vi "backup_imp_test_v8.vi"() -> ()   [LabVIEW 2014]
uses:
  <vilib>/eio/EIOPropertyNode/EIOPropertyNode.xnode
  <vilib>/LabVIEW Targets/FPGA/cRIO/shared/nicrio_ModuleControls/nicrio_cRIO-9237_DataRatesRing.ctl
  <vilib>/LabVIEW Targets/FPGA/cRIO/shared/nicrio_ModuleControls/nicrio_cRIO-9237_ExcitationVoltageRing.ctl
  <vilib>/rvi/eio/common/nirviEmuTemplatePropertyGet_errors.vi
  <vilib>/rvi/eio/common/nirviEmuTemplatePropertyGet_noerrors.vi
  <vilib>/rvi/eio/common/nirviEmuTemplatePropertySet_errors.vi
  <vilib>/rvi/eio/common/nirviEmuTemplatePropertySet_noerrors.vi
  <vilib>/eio/EIONode/EIONode.xnode
  <vilib>/rvi/eio/common/nirviEmuTemplateMethod_errors.vi
  <vilib>/rvi/Analysis/measure/butterworth/XNode/niFpgaButterworthFilter.xnode
  <vilib>/rvi/DataTransferAndStorage/Container/XNode/niFpgaContainer.xnode
  <vilib>/rvi/FXPMathLib/FxpMul/XNode/nifxpmath_Multiplier.xnode
  <vilib>/rvi/FXPMathLib/sim/FxpSim.dll
  <vilib>/rvi/FXPMathLib/FxpSinAndCos/XNode/nifxpmath_SinAndCos.xnode
  <vilib>/rvi/FXPMathLib/FxpSinAndCos/simVIs/DllFxpSinAndCosTemp_sub.vi
  <vilib>/rvi/FXPMathLib/FxpSinAndCos/subVIs/nifxpmath_SinAndCos_SimConfig.ctl
  <vilib>/rvi/FXPMathLib/FxpSub/XNode/nifxpmath_Sub.xnode
  <vilib>/rvi/FXPMathLib/FxpAdd/XNode/nifxpmath_Add.xnode
  <vilib>/rvi/interface/RandomDataEmulation/nirviRandomDataFpgaMultiElementTemplate.vi
panel:
  out "omega_y (rad/s)":fxp<+/-,36,13>
  out "Dy_d (mm/s)":fxp<+/-,36,13>
  in  "Vy. Est.":i16(ring) items=["T", "Mavg"]
  out "omega_y (Mavg)":fxp<+/-,36,13>
  out "Dy_d (Mavg)":fxp<+/-,36,13>
  in  "Dy_d_M_avg_Tc (uSec)":i32 caption="Dp_d_M_avg_Tc (uSec)"
  out "Dp_d (Mavg)":fxp<+/-,36,13>
  out "omega_p (Mavg)":fxp<+/-,36,13>
  in  "Dp_d_M_avg_Tc (uSec)":i32
  out "Dp_d (T)":fxp<+/-,36,13>
  out "omega_p (T)":fxp<+/-,36,13>
  in  "Vp. Est.":i16(ring) items=["T", "Mavg"]
  in  "Mag. factor":fxp<+/-,20,3>
  in  "Mag. encoder_p":bool
  in  "Belt_op":fxp<+/-,7,7>
  in  "Belt_mp":fxp<+/-,6,6>
  in  "Belt_oy":fxp<+/-,7,7>
  in  "Belt_my":fxp<+/-,6,6>
  out "Fp_dc":fxp<+/-,32,10>
  out "Fy_dc":fxp<+/-,32,10>
  in  "Zero_y":bool
  in  "Zero_p":bool
  in  "mt0_omega_p":u32
  in  "Encoder reset":bool
  out "fpt_d":fxp<+/-,36,18>
  out "Dp_error_dd":fxp<+/-,36,16>
  out "Dp_error_d":fxp<+/-,33,8>
  in  "Dp_dd coeff.":i32[](array[numeric])=[946630756, 63555534]
  out "Dp_dd":fxp<+/-,36,25>
  out "dFp_PID":fxp<+/-,36,18>
  in  "dFp_PID coeff.":i32[](array[numeric])=[946630756, 63555534]
  out "fpt_i":fxp<+/-,34,18>
  in  "Bv_p":fxp<+/-,22,8>
  in  "Kv_p":fxp<+/-,22,8>
  out "Dp_error":fxp<+/-,22,7>
  out "Dpr_sin":fxp<+/-,22,7>
  in  "Sin offset_p":fxp<+/-,22,7>
  in  "Sin magnitude_p":fxp<+/-,21,6>
  out "Dpr_sin_dd":fxp<+/-,35,20>
  out "Dpr_sin_d":fxp<+/-,33,15>
  out "Sin omega_p":fxp<+/-,34,9>
  in  "Sin wave freq._p (Hz)":fxp<+/-,32,6>
  in  "Dpr_step":fxp<+/-,22,7>
  out "Dpr_for":fxp<+/-,22,7>
  in  "Command_p":i16(ring) items=["Step", "Sine"]
  in  "Ki_p":fxp<+/-,36,9>
  out "Fp_PID":fxp<+/-,36,16>
  in  "fp_tolorance":fxp<+,22,6>
  out "fp_tilde":fxp<+/-,33,10>
  in  "Kd_p":fxp<+/-,36,9>
  in  "Kp_p":fxp<+/-,36,9>
  out "Fr_p":fxp<+/-,32,10>
  in  "S/F coeff_p":fxp<+/-,25,-10>
  in  "S/F coeff_y":fxp<+/-,25,-10>
  out "va_p":fxp<+/-,36,7>
  out "vb_p":fxp<+/-,37,8>
  out "vq_p_F":fxp<+/-,20,5> format="%.57g"
  out "vd_p_F":fxp<+/-,20,5>
  in  "dFp_add":bool
  in  "Stop motor_p":bool
  out "Force_p":fxp<+/-,32,10>
  in  "Strain selection_p":i16(ring) items=["Raw", "Avg.8", "Avg.8 w. filter"]
  out "Strain_p (Avg8 w. f)":fxp<+/-,36,8>
  in  "Strain_p Avg.8 coeff.":i32[](array[numeric])=[946630756, 63555534]
  out "Strain_p (Avg8)":fxp<+/-,36,4>
  out "Raw Strain_p":fxp<+/-,36,4>
  out "Mod6/AI3":fxp<+/-,36,4>
  in  "Strain gage reset_p":bool
  out "Dp_d (mm/s)":fxp<+/-,36,13>
  out "omega_p (rad/s)":fxp<+/-,36,13>
  out "mt_omega_p":u32
  out "rad_p(NrTheta)":fxp<+/-,33,20>
  out "D_p(mm)":fxp<+/-,32,7>
  out "Encoder Position_p":i32
  in  "Encoder reset_p":bool
  out "Strain_y (Avg8 w. f)":fxp<+/-,36,8>
  in  "Strain_y Avg8 coeff.":i32[](array[numeric])=[-898916953, 1957103773, 3888751]
  out "Dyr_for":fxp<+/-,22,7>
  in  "Command_y":i16(ring) items=["Step", "Sine"]
  out "Strain_y (Avg8)":fxp<+/-,36,4>
  in  "Strain selection_y":i16(ring) items=["Raw", "Avg.8", "Avg.8 w. filter"]
  out "vb_y":fxp<+/-,38,8>
  out "va_y":fxp<+/-,38,8>
  out "fyt_d":fxp<+/-,36,18>
  out "Fr_y":fxp<+/-,32,10>
  in  "Bv_y":fxp<+/-,22,8>
  out "Dy_error_dd":fxp<+/-,36,16>
  out "Dy_error_d":fxp<+/-,33,8>
  in  "Kv_y":fxp<+/-,22,8>
  out "Dy_error":fxp<+/-,22,7>
  out "Dyr_sin_dd":fxp<+/-,35,20>
  out "Dyr_sin_d":fxp<+/-,33,15>
  out "Sin omega_y":fxp<+/-,34,9>
  out "Dyr_sin":fxp<+/-,22,7>
  in  "Sin offset_y":fxp<+/-,22,7>
  in  "Sin magnitude_y":fxp<+/-,21,6>
  out "Time now(s)":fxp<+,52,14>
  in  "Sin wave freq._y (Hz)":fxp<+/-,32,6>
  in  "Dyr_step":fxp<+/-,22,7>
  in  "Drive mode":i16(ring) items=["Backward", "Forward"]
  out "Dy_dd":fxp<+/-,36,25>
  in  "Dy_dd coeff.":i32[](array[numeric])=[946630756, 63555534]
  out "dFy_PID":fxp<+/-,36,18>
  in  "dFy_PID coeff.":i32[](array[numeric])=[946630756, 63555534]
  out "fyt_i":fxp<+/-,36,16>
  out "Fy_PID":fxp<+/-,36,16>
  in  "fy_tolorance":fxp<+,22,6>
  in  "Ki_y":fxp<+/-,36,9>
  in  "Kd_y":fxp<+/-,36,9>
  out "fy_tilde":fxp<+/-,32,10>
  in  "Kp_y":fxp<+/-,36,9>
  out "vq_y_F":fxp<+/-,20,5> format="%.57g"
  out "vd_y_F":fxp<+/-,20,5>
  in  "dFy_add":bool
  in  "Stop motor_y":bool
  out "Dy_d (T)":fxp<+/-,36,13>
  out "omega_y (T)":fxp<+/-,36,13>
  in  "mt0_omega_y":u32
  out "mt_omega_y":u32
  out "rad_y(NrTheta)":fxp<+/-,33,20>
  out "D_y(mm)":fxp<+/-,32,7>
  out "Encoder Position_y":i32
  in  "Encoder reset_y":bool
  in  "Ini coe.":bool
  out "Loop rate (kHz)":fxp<+/-,36,7>
  out "Force_y":fxp<+/-,32,10>
  out "Raw Strain_y":fxp<+/-,36,4>
  in  "Strain gage reset_y":bool
  in  "Stop (Strain)":bool
  out "Mod6/AI2":fxp<+/-,36,4>
  in  "Excitation Voltage":T1 items=["2.5 Volts", "3.3 Volts", "5.0 Volts", "10.0 Volts", "External Excitation"]
  in  "Data Rate":T2=1 items=["50.000 kS/s (NI 9237)"=1, "25.000 kS/s (NI 9237)"=2, "16.667 kS/s (NI 9237)"=3, "12.500 kS/s (NI 9237)"=4, "10.000 kS/s (NI 9237)"=5, "8.333 kS/s (NI 9237)"=6, "7.143 kS/s (NI 9237)"=7, "6.250 kS/s (NI 9237)"=8, "5.556 kS/s (NI 9237)"=9, "5.000 kS/s (NI 9237)"=10, "4.545 kS/s (NI 9237)"=11, "4.167 kS/s (NI 9237)"=12, "3.846 kS/s (NI 9237)"=13, "3.571 kS/s (NI 9237)"=14, "3.333 kS/s (NI 9237)"=15, "3.125 kS/s (NI 9237)"=16, "2.941 kS/s (NI 9237)"=17, "2.778 kS/s (NI 9237)"=18, "2.632 kS/s (NI 9237)"=19, "2.500 kS/s (NI 9237)"=20, "2.381 kS/s (NI 9237)"=21, "2.273 kS/s (NI 9237)"=22, "2.174 kS/s (NI 9237)"=23, "2.083 kS/s (NI 9237)"=24, "2.000 kS/s (NI 9237)"=25, "1.923 kS/s (NI 9237)"=26, "1.852 kS/s (NI 9237)"=27, "1.786 kS/s (NI 9237)"=28, "1.724 kS/s (NI 9237)"=29, "1.667 kS/s (NI 9237)"=30, "1.613 kS/s (NI 9237)"=31]
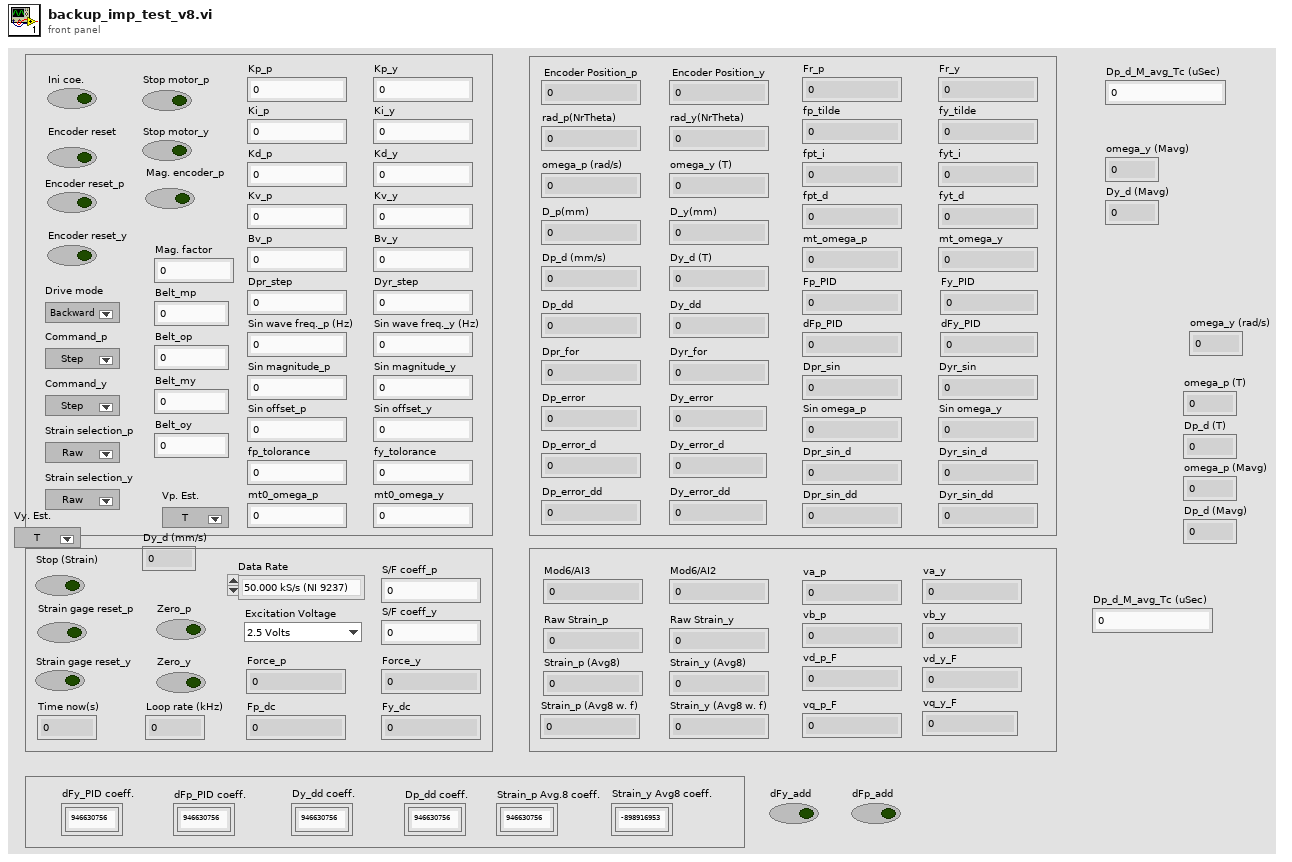
[diagram p1: front panel]
types:
  T1 = typedef "nicrio_cRIO-9237_ExcitationVoltageRing.ctl" = u8
  T2 = typedef "nicrio_cRIO-9237_DataRatesRing.ctl" = u8
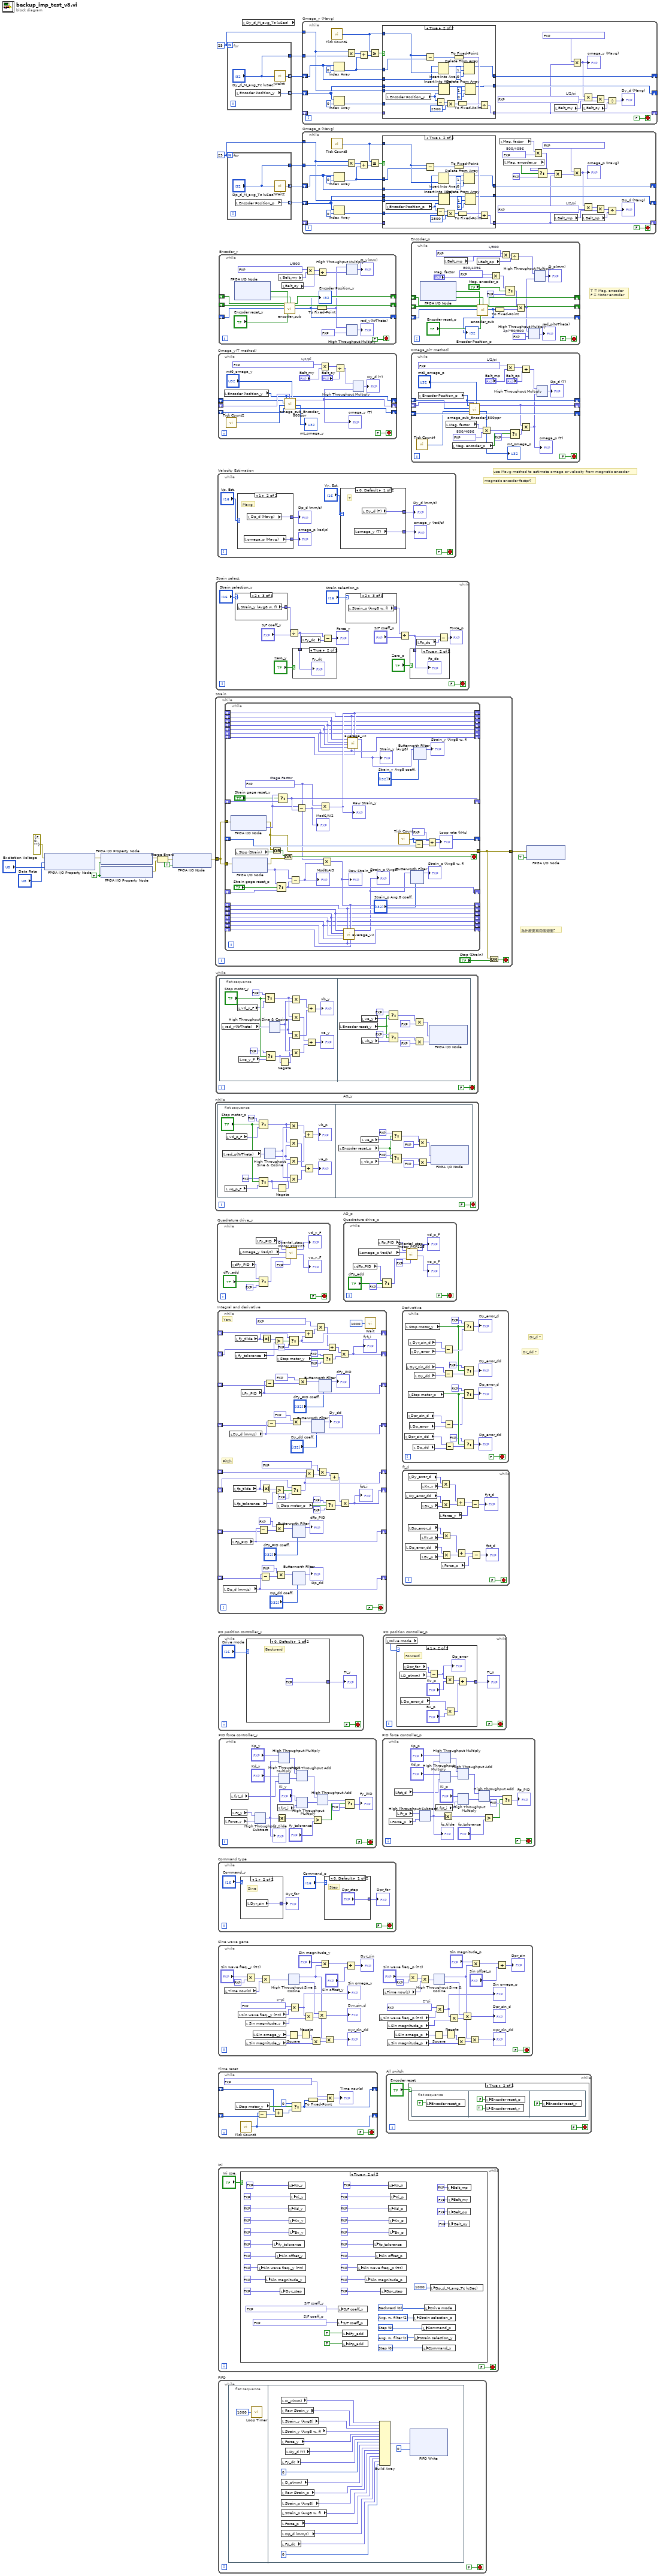
[diagram p0: block diagram]
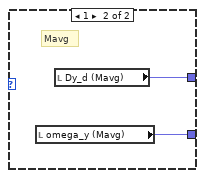
[diagram p4: hidden frame]
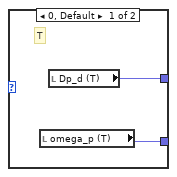
[diagram p5: hidden frame]
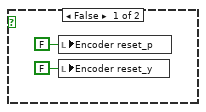
[diagram p6: hidden frame]
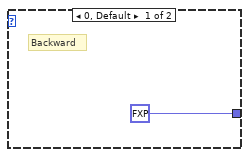
[diagram p7: hidden frame]
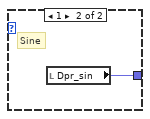
[diagram p8: hidden frame]
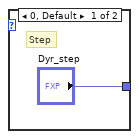
[diagram p9: hidden frame]
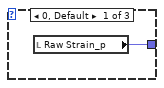
[diagram p12: hidden frame]
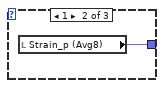
[diagram p13: hidden frame]
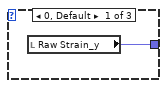
[diagram p14: hidden frame]
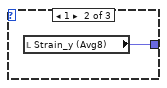
[diagram p15: hidden frame]
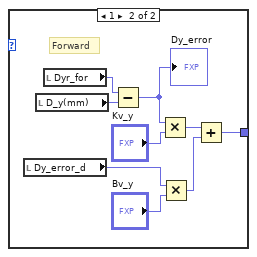
[diagram p16: hidden frame]
diagram:
  w5 = 25
  w8 = 25
  w13 = TRUE ("Half-Bridge Enable")
  # "use Mavg method to estimate omega or velocity from magnetic encoder"
  # "T = Mag. encoder\nF = Motor encoder"
  # "magnetic encoder factpr?"
  # "為什麼要寫兩個迴圈?"
  # "Dr_dd ?"
  # "Dr_d ?"
  n1 = xnode "FPGA I/O Property Node"("error in"=errorcluster {"status"=FALSE, "code"=0, "source"=""}, "Data Rate"="Data Rate", "Excitation Voltage"="Excitation Voltage") -> ("error out"=w18:errorcluster)  [unwired: 1 in, 1 out]
  n2 = xnode "FPGA I/O Property Node"("error in"=w18, "Half-Bridge Enable"=w13) -> ("error out"=w11:errorcluster)  [unwired: 1 in, 1 out]
  n3 = xnode "FPGA I/O Property Node"("Half-Bridge Enable"=w13) -> ("error out"=w10:errorcluster)  [unwired: 2 in, 1 out]
  n4 = Merge Errors(w11, w10) -> (w12:errorcluster)
  n5 = xnode "FPGA I/O Node"("error in"=w12, "Mod6/Start"=TRUE) -> ("error out"=w16:errorcluster)  [unwired: 1 in, 1 out]
  n6 = while "Strain" {
    tunnel: w16 -> [w23]
    tunnel: [w21] -> w9
    stop <- w22 stop-if-true
    n7 = while {
      tunnel: w23 -> [w69]
      tunnel: [w42] -> w21
      shift-right: [w66] -> _
      shift-left: _ -> [w67]
      shift-right: [w62] -> _
      shift-left: _ -> [w63]
      shift-right: [w57] -> _
      shift-left: _ -> [w56]
      shift-right: [w56] -> _
      shift-left: _ -> [w55]
      shift-right: [w55] -> _
      shift-left: _ -> [w54]
      shift-right: [w54] -> _
      shift-left: _ -> [w53]
      shift-right: [w53] -> _
      shift-left: _ -> [w52]
      shift-right: [w52] -> _
      shift-left: _ -> [w51]
      shift-right: [w51] -> _
      shift-left: _ -> [w50]
      tunnel: w23 -> [w46]
      shift-right: [w39] -> _
      shift-left: _ -> [w40]
      shift-right: [w35] -> _
      shift-left: _ -> [w34]
      shift-right: [w34] -> _
      shift-left: _ -> [w33]
      shift-right: [w33] -> _
      shift-left: _ -> [w32]
      shift-right: [w32] -> _
      shift-left: _ -> [w31]
      shift-right: [w31] -> _
      shift-left: _ -> [w30]
      shift-right: [w30] -> _
      shift-left: _ -> [w29]
      shift-right: [w29] -> _
      shift-left: _ -> [w28]
      stop <- w43 stop-if-true
      w37 = fxp<+,20,2> 2.115001678466797  # Gage Factor
      n8 = xnode "FPGA I/O Node"("error in"=w69) -> ("error out"=w42:errorcluster, "Mod6/AI2"=w64:fxp<+/-,24,-4>)  [unwired: 1 in, 1 out]
      n9 = xnode "FPGA I/O Node"("error in"=w46) -> ("error out"=w44:errorcluster, "Mod6/AI3"=w38:fxp<+/-,24,-4>)  [unwired: 1 in, 1 out]
      n10 = local read "Stop (Strain)"() -> (w68:bool)
      n11 = Or(x=w42, y=w68) -> (x .or. y?=w45:bool)
      n12 = Select(t=w38, s="Strain gage reset_p", f=w40) -> (s? t:f=w39:fxp<+/-,24,-4>)
      n13 = Select(t=w64, s="Strain gage reset_y", f=w67) -> (s? t:f=w66:fxp<+/-,24,-4>)
      n14 = Or(x=w45, y=w44) -> (x .or. y?=w43:bool)
      n15 = Subtract(x=w38, y=w39) -> (x-y=w36:fxp<+/-,30,-3>)
      "Mod6/AI3" <- w36
      n16 = Subtract(x=w64, y=w66) -> (x-y=w65:fxp<+/-,30,-3>)
      "Mod6/AI2" <- w65
      n17 = Multiply(x=w37, y=w65) -> (x*y=w57:fxp<+/-,41,6>)
      "Raw Strain_y" <- w57
      n18 = Multiply(x=w37, y=w36) -> (x*y=w35:fxp<+/-,50,-1>)
      "Raw Strain_p" <- w35
      n19 = call "average_v2.vi"("Numeric 8"=w28, "Numeric"=w35, "Numeric 7"=w29, "Numeric 2"=w34, "Numeric 6"=w30, "Numeric 5"=w31, "Numeric 4"=w32, "Numeric 3"=w33) -> ("Mean (8pt)"=w27:fxp<+/-,32,4>)  [unwired: 1 in, 2 out]
      "Strain_p (Avg8)" <- w27
      n20 = call "average_v2.vi"("Numeric 8"=w50, "Numeric"=w57, "Numeric 7"=w51, "Numeric 2"=w56, "Numeric 6"=w52, "Numeric 5"=w53, "Numeric 4"=w54, "Numeric 3"=w55) -> ("Mean (8pt)"=w49:fxp<+/-,32,4>)  [unwired: 1 in, 2 out]
      "Strain_y (Avg8)" <- w49
      n21 = call "Tick Count"() -> ("Tick Count(uSec)"=w62:u32)
      n22 = xnode "Butterworth Filter"("input data"=w27, "scaled coefficients"="Strain_p Avg.8 coeff.") -> ("output data"=→"Strain_p (Avg8 w. f)":fxp<+/-,36,8>)  [unwired: 1 in]
      n23 = xnode "Butterworth Filter"("input data"=w49, "scaled coefficients"="Strain_y Avg8 coeff.") -> ("output data"=→"Strain_y (Avg8 w. f)":fxp<+/-,32,4>)  [unwired: 1 in]
      n24 = Subtract(x=w62, y=w63) -> (x-y=w60:fxp<+/-,32,16>)
      n25 = Divide(x=fxp<+,7,10> 1000.0, y=w60) -> (x/y=→"Loop rate (kHz)":fxp<+/-,40,27>)
    }
    n26 = Or(x=w21, y="Stop (Strain)") -> (x .or. y?=w22:bool)
  }
  n27 = while "AO_p" {
    stop <- FALSE stop-if-true
    n28 = flat-sequence {
      frame #0 {
        n29 = local read "rad_p(NrTheta)"() -> (w98:fxp<+/-,33,20>)
        n30 = local read "vq_p_F"() -> (w99:fxp<+/-,20,5>)
        n31 = local read "vd_p_F"() -> (w101:fxp<+/-,20,5>)
        n32 = Select(t=fxp<+/-,20,5> 0.0, s="Stop motor_p", f=w101) -> (s? t:f=w90:fxp<+/-,20,5>)
        n33 = Select(t=fxp<+,1,1> 0.0, s="Stop motor_p", f=w99) -> (s? t:f=w89:fxp<+/-,20,5>)
        n34 = xnode "High Throughput Sine & Cosine"("x (pi)"=w98) -> ("sin(x)"=w92:fxp<+/-,16,2>, "cos(x)"=w91:fxp<+/-,16,2>)
        n35 = Negate(x=w89) -> (-x=w97:fxp<+/-,21,6>)
        n36 = Multiply(x=w90, y=w92) -> (x*y=w96:fxp<+/-,36,7>)
        n37 = Multiply(x=w90, y=w91) -> (x*y=w94:fxp<+/-,36,7>)
        n38 = Multiply(x=w91, y=w89) -> (x*y=w95:fxp<+/-,36,7>)
        n39 = Multiply(x=w92, y=w97) -> (x*y=w93:fxp<+/-,35,6>)
        n40 = Add(x=w96, y=w95) -> (x+y=→"vb_p":fxp<+/-,37,8>)
        n41 = Add(x=w94, y=w93) -> (x+y=→"va_p":fxp<+/-,36,7>)
      }
      frame #1 {
        n42 = local read "Encoder reset_p"() -> (w134:bool)
        n43 = local read "vb_p"() -> (w135:fxp<+/-,37,8>)
        n44 = local read "va_p"() -> (w136:fxp<+/-,36,7>)
        n45 = Select(t=fxp<+,2,2> 3.0, s=w134, f=w136) -> (s? t:f=w142:fxp<+/-,36,7>)
        n46 = Select(t=fxp<+,1,1> 0.0, s=w134, f=w135) -> (s? t:f=w141:fxp<+/-,37,8>)
        n47 = Multiply(x=w142, y=fxp<+/-,1,0> -0.5) -> (x*y=w137:fxp<+/-,36,6>)
        n48 = Multiply(x=w141, y=fxp<+/-,1,0> -0.5) -> (x*y=w138:fxp<+/-,36,6>)
        n49 = xnode "FPGA I/O Node"("Mod8/AO0"=w137, "Mod8/AO1"=w138) -> ()  [unwired: 2 in, 2 out]
      }
    }
  }
  n50 = while "AO_y" {
    stop <- FALSE stop-if-true
    n51 = flat-sequence {
      frame #0 {
        n52 = local read "rad_y(NrTheta)"() -> (w162:fxp<+/-,33,20>)
        n53 = local read "vd_y_F"() -> (w160:fxp<+/-,20,5>)
        n54 = local read "vq_y_F"() -> (w159:fxp<+/-,20,5>)
        n55 = Select(t=fxp<+/-,20,5> 0.0, s="Stop motor_y", f=w160) -> (s? t:f=w154:fxp<+/-,20,5>)
        n56 = Select(t=fxp<+/-,20,5> 0.0, s="Stop motor_y", f=w159) -> (s? t:f=w153:fxp<+/-,20,5>)
        n57 = xnode "High Throughput Sine & Cosine"("x (pi)"=w162) -> ("sin(x)"=w156:fxp<+/-,17,2>, "cos(x)"=w155:fxp<+/-,17,2>)
        n58 = Negate(x=w153) -> (-x=w152:fxp<+/-,21,6>)
        n59 = Multiply(x=w154, y=w156) -> (x*y=w151:fxp<+/-,37,7>)
        n60 = Multiply(x=w154, y=w155) -> (x*y=w149:fxp<+/-,37,7>)
        n61 = Multiply(x=w155, y=w153) -> (x*y=w150:fxp<+/-,37,7>)
        n62 = Multiply(x=w156, y=w152) -> (x*y=w148:fxp<+/-,36,6>)
        n63 = Add(x=w151, y=w150) -> (x+y=→"vb_y":fxp<+/-,38,8>)
        n64 = Add(x=w149, y=w148) -> (x+y=→"va_y":fxp<+/-,37,7>)
      }
      frame #1 {
        n65 = local read "Encoder reset_y"() -> (w195:bool)
        n66 = local read "va_y"() -> (w194:fxp<+/-,38,8>)
        n67 = local read "vb_y"() -> (w193:fxp<+/-,38,8>)
        n68 = Select(t=fxp<+,2,2> 3.0, s=w195, f=w194) -> (s? t:f=w199:fxp<+/-,38,8>)
        n69 = Select(t=fxp<+,1,1> 0.0, s=w195, f=w193) -> (s? t:f=w198:fxp<+/-,38,8>)
        n70 = Multiply(x=w199, y=fxp<+/-,1,0> -0.5) -> (x*y=w202:fxp<+/-,39,8>)
        n71 = Multiply(x=w198, y=fxp<+/-,1,0> -0.5) -> (x*y=w203:fxp<+/-,37,6>)
        n72 = xnode "FPGA I/O Node"("Mod8/AO2"=w202, "Mod8/AO3"=w203) -> ()  [unwired: 2 in, 2 out]
      }
    }
  }
  n73 = while "Strain select." {
    stop <- FALSE stop-if-true
    n74 = case shown="2" "Strain selection_y" {
      tunnel: [w224 w225 w226] -> w217
      frame 0, Default {
        n75 = local read "Raw Strain_y"() -> (w224:fxp<+/-,36,4>)
      }
      frame 1 {
        n76 = local read "Strain_y (Avg8)"() -> (w225:fxp<+/-,36,4>)
      }
      frame 2 {
        n77 = local read "Strain_y (Avg8 w. f)"() -> (w226:fxp<+/-,36,8>)
      }
    }
    n78 = Divide(x=w217, y="S/F coeff_y") -> (x/y=w210:fxp<+/-,32,10>)
    n79 = case shown="True" "Zero_y" {
      tunnel: w210 -> [_ w220]
      frame False {
      }
      frame True {
        "Fy_dc" <- w220
      }
    }
    n80 = local read "Fy_dc"() -> (w211:fxp<+/-,32,10>)
    n81 = Subtract(x=w210, y=w211) -> (x-y=→"Force_y":fxp<+/-,33,11>)
    n82 = case shown="2" "Strain selection_p" {
      tunnel: [w221 w222 w223] -> w215
      frame 0, Default {
        n83 = local read "Raw Strain_p"() -> (w221:fxp<+/-,36,4>)
      }
      frame 1 {
        n84 = local read "Strain_p (Avg8)"() -> (w222:fxp<+/-,36,4>)
      }
      frame 2 {
        n85 = local read "Strain_p (Avg8 w. f)"() -> (w223:fxp<+/-,36,8>)
      }
    }
    n86 = Divide(x=w215, y="S/F coeff_p") -> (x/y=w207:fxp<+/-,32,10>)
    n87 = case shown="True" "Zero_p" {
      tunnel: w207 -> [_ w219]
      frame False {
      }
      frame True {
        "Fp_dc" <- w219
      }
    }
    n88 = local read "Fp_dc"() -> (w205:fxp<+/-,32,10>)
    n89 = Subtract(x=w207, y=w205) -> (x-y=→"Force_p":fxp<+/-,33,11>)
  }
  n90 = while "Quadrature drive_y" {
    stop <- FALSE stop-if-true
    n91 = local read "dFy_PID"() -> (w228:fxp<+/-,36,18>)
    n92 = local read "omega_y (rad/s)"() -> (w236:fxp<+/-,36,13>)
    n93 = local read "Fy_PID"() -> (w229:fxp<+/-,36,16>)
    n94 = Select(t=w228, s="dFy_add", f=fxp<+,1,1> 0.0) -> (s? t:f=w232:fxp<+/-,36,18>)
    n95 = call "Oriental_step_motor_PKP225.vi"("F_Threshold"=fxp<+,12,12> 10.0, "dFmr"=w232, "omega"=w236, "Fmr"=w229) -> ("vq_F"=→"vq_y_F":fxp<+/-,20,5>, "vd_F"=→"vd_y_F":fxp<+/-,20,5>)  [unwired: 6 in]
  }
  n96 = while "Integral and derivative" {
    shift-right: [w292] -> _
    shift-left: _ -> [w291]
    shift-right: [w284] -> _
    shift-left: _ -> [w283]
    shift-right: [w294] -> _
    shift-left: _ -> [w295]
    shift-right: [w274] -> _
    shift-left: _ -> [w273]
    shift-right: [w260] -> _
    shift-left: _ -> [w263]
    shift-right: [w253] -> _
    shift-left: _ -> [w252]
    shift-right: [w247] -> _
    shift-left: _ -> [w246]
    shift-right: [w242] -> _
    shift-left: _ -> [w243]
    stop <- FALSE stop-if-true
    # "Pitch"
    # "Yaw"
    n97 = local read "Dp_d (mm/s)"() -> (w242:fxp<+/-,36,13>)
    n98 = local read "Dy_d (mm/s)"() -> (w274:fxp<+/-,36,13>)
    n99 = local read "Fp_PID"() -> (w247:fxp<+/-,36,16>)
    n100 = local read "fp_tilde"() -> (w264:fxp<+/-,33,10>)
    n101 = local read "fp_tolorance"() -> (w267:fxp<+,22,6>)
    n102 = local read "fy_tolorance"() -> (w270:fxp<+,22,6>)
    n103 = local read "fy_tilde"() -> (w296:fxp<+/-,32,10>)
    n104 = local read "Fy_PID"() -> (w294:fxp<+/-,36,16>)
    n105 = Subtract(x=w247, y=w246) -> (x-y=w251:fxp<+/-,37,17>)
    n106 = Subtract(x=w242, y=w243) -> (x-y=w244:fxp<+/-,37,14>)
    n107 = Absolute Value(x=w264) -> (abs(x)=w268:fxp<+,33,10>)
    n108 = Absolute Value(x=w296) -> (abs(x)=w298:fxp<+,32,10>)
    n109 = Subtract(x=w294, y=w295) -> (x-y=w282:fxp<+/-,37,17>)
    n110 = Subtract(x=w274, y=w273) -> (x-y=w276:fxp<+/-,36,11>)
    n111 = Greater?(x=w298, y=w270) -> (0:w299:bool)
    n112 = Greater?(x=w268, y=w267) -> (0:w266:bool)
    n113 = Multiply(x=fxp<+,7,10> 1000.0, y=w251) -> (x*y=w249:fxp<+/-,32,18>)
    n114 = Multiply(x=fxp<+,7,10> 1000.0, y=w244) -> (x*y=w240:fxp<+/-,36,21>)
    n115 = local read "Stop motor_y"() -> (w285:bool)
    n116 = local read "Stop motor_p"() -> (w255:bool)
    n117 = Select(t=w296, s=w299, f=fxp<+/-,33,11> 0.0) -> (s? t:f=w292:fxp<+/-,33,11>)
    n118 = Select(t=w264, s=w266, f=fxp<+,1,1> 0.0) -> (s? t:f=w260:fxp<+/-,33,10>)
    n119 = Multiply(x=fxp<+,7,10> 1000.0, y=w276) -> (x*y=w275:fxp<+/-,36,21>)
    n120 = xnode "Butterworth Filter"("input data"=w249, "scaled coefficients"="dFp_PID coeff.") -> ("output data"=→"dFp_PID":fxp<+/-,36,22>)  [unwired: 1 in]
    n121 = xnode "Butterworth Filter"("input data"=w240, "scaled coefficients"="Dp_dd coeff.") -> ("output data"=→"Dp_dd":fxp<+/-,36,25>)  [unwired: 1 in]
    n122 = Multiply(x=fxp<+,7,10> 1000.0, y=w282) -> (x*y=w279:fxp<+/-,32,18>)
    n123 = Add(x=w291, y=w292) -> (x+y=w297:fxp<+/-,34,12>)
    n124 = Multiply(x=w263, y=w260) -> (x*y=w262:fxp<+/-,34,12>)
    n125 = xnode "Butterworth Filter"("input data"=w275, "scaled coefficients"="Dy_dd coeff.") -> ("output data"=→"Dy_dd":fxp<+/-,36,25>)  [unwired: 1 in]
    n126 = Multiply(x=fxp<+/-,30,12> 0.000499725341796875, y=w297) -> (x*y=w290:fxp<+/-,34,10>)
    n127 = Multiply(x=fxp<+/-,30,12> 0.000499725341796875, y=w262) -> (x*y=w259:fxp<+/-,34,10>)
    n128 = xnode "Butterworth Filter"("input data"=w279, "scaled coefficients"="dFy_PID coeff.") -> ("output data"=→"dFy_PID":fxp<+/-,36,22>)  [unwired: 1 in]
    n129 = Select(t=fxp<+,1,1> 0.0, s=w285, f=fxp<+,1,1> 1.0) -> (s? t:f=w288:fxp<+,1,1>)
    n130 = Select(t=fxp<+,1,1> 0.0, s=w255, f=fxp<+,1,1> 1.0) -> (s? t:f=w257:fxp<+,1,1>)
    n131 = Add(x=w290, y=w283) -> (x+y=w289:fxp<+/-,36,16>)
    n132 = Add(x=w259, y=w252) -> (x+y=w258:fxp<+/-,36,16>)
    n133 = Multiply(x=w289, y=w288) -> (x*y=w284:fxp<+/-,34,18>)
    "fyt_i" <- w284
    n134 = Multiply(x=w258, y=w257) -> (x*y=w253:fxp<+/-,34,18>)
    "fpt_i" <- w253
    n135 = call "Wait"("Count(uSec)"=u32 1000) -> ()  [unwired: 1 out]
  }
  n136 = while "Velocity Estimation" {
    stop <- FALSE stop-if-true
    n137 = case shown="1" "Vp. Est." {
      tunnel: [w345 w346] -> w338
      tunnel: [w344 w347] -> w337
      frame 0, Default {
        # "T"
        n138 = local read "omega_p (T)"() -> (w345:fxp<+/-,36,13>)
        n139 = local read "Dp_d (T)"() -> (w344:fxp<+/-,36,13>)
      }
      frame 1 {
        # "Mavg"
        n140 = local read "omega_p (Mavg)"() -> (w346:fxp<+/-,36,13>)
        n141 = local read "Dp_d (Mavg)"() -> (w347:fxp<+/-,36,13>)
      }
    }
    "Dp_d (mm/s)" <- w337
    "omega_p (rad/s)" <- w338
    n142 = case shown="0, Default" "Vy. Est." {
      tunnel: [w341 w343] -> w335
      tunnel: [w340 w342] -> w334
      frame 0, Default {
        # "T"
        n143 = local read "omega_y (T)"() -> (w340:fxp<+/-,36,13>)
        n144 = local read "Dy_d (T)"() -> (w341:fxp<+/-,36,13>)
      }
      frame 1 {
        # "Mavg"
        n145 = local read "omega_y (Mavg)"() -> (w342:fxp<+/-,36,13>)
        n146 = local read "Dy_d (Mavg)"() -> (w343:fxp<+/-,36,13>)
      }
    }
    "Dy_d (mm/s)" <- w335
    "omega_y (rad/s)" <- w334
  }
  n147 = while "Omega_y(T method)" {
    shift-right: [w355] -> _
    shift-left: _ -> [w356]
    shift-right: [w349] -> _
    shift-left: _ -> [w359]
    shift-right: [w361] -> _
    shift-left: _ -> [w362]
    stop <- FALSE stop-if-true
    w354 = fxp<+/-,32,0> 0.3183098859153688  # L/2/pi
    n148 = local read "Encoder Position_y"() -> (w355:i32)
    n149 = call "Tick Count2"() -> ("Tick Count(Ticks)"=w363:u32)
    n150 = call "omega_sub_Encoder_800ppr.vi"("mt0"="mt0_omega_y", "omega_pre"=w359, "ticks_m_pre"=w362, "ticks"=w363, "count_pre"=w356, "count"=w355) -> ("ticks_m"=w361:u32, "mt"=→"mt_omega_y":u32, "omega"=w349:fxp<+/-,36,13>)  [unwired: 3 in]
    "omega_y (T)" <- w349
    n151 = Multiply(x=w354, y="Belt_my") -> (x*y=w352:fxp<+/-,38,6>)
    n152 = Divide(x=w352, y="Belt_oy") -> (x/y=w350:fxp<+/-,20,1>)
    n153 = xnode ("High Throughput Multiply")("x"=w350, "y"=w349) -> ("x*y"=→"Dy_d (T)":fxp<+/-,56,14>)
  }
  n154 = while "PD position controller_y" {
    stop <- FALSE stop-if-true
    n155 = case shown="0, Default" "Drive mode" {
      tunnel: [fxp<+/-,62,19> 0.0 w369] -> w365
      frame 0, Default {
        # "Backward"
      }
      frame 1 {
        # "Forward"
        n156 = local read "Dy_error_d"() -> (w371:fxp<+/-,33,8>)
        n157 = local read "D_y(mm)"() -> (w376:fxp<+/-,32,7>)
        n158 = local read "Dyr_for"() -> (w368:fxp<+/-,22,7>)
        n159 = Subtract(x=w368, y=w376) -> (x-y=w375:fxp<+/-,33,8>)
        "Dy_error" <- w375
        n160 = Multiply(x=w375, y="Kv_y") -> (x*y=w373:fxp<+/-,54,15>)
        n161 = Multiply(x=w371, y="Bv_y") -> (x*y=w370:fxp<+/-,55,16>)
        n162 = Add(x=w373, y=w370) -> (x+y=w369:fxp<+/-,55,16>)
      }
    }
    "Fr_y" <- w365
  }
  n163 = while "Command type" {
    stop <- FALSE stop-if-true
    n164 = case shown="1" "Command_y" {
      tunnel: ["Dyr_step" w385] -> w380
      frame 0, Default {
        # "Step"
      }
      frame 1 {
        # "Sine"
        n165 = local read "Dyr_sin"() -> (w385:fxp<+/-,22,7>)
      }
    }
    "Dyr_for" <- w380
    n166 = case shown="0, Default" "Command_p" {
      tunnel: ["Dpr_step" w383] -> w378
      frame 0, Default {
        # "Step"
      }
      frame 1 {
        # "Sine"
        n167 = local read "Dpr_sin"() -> (w383:fxp<+/-,22,7>)
      }
    }
    "Dpr_for" <- w378
  }
  n168 = while "Sine wave gene" {
    stop <- FALSE stop-if-true
    w391 = fxp<+,20,3> 6.2831878662109375  # 2*pi
    w423 = fxp<+,20,3> 6.2831878662109375  # 2*pi
    n169 = local read "Time now(s)"() -> (w429:fxp<+,52,14>)
    n170 = local read "Sin wave freq._y (Hz)"() -> (w422:fxp<+/-,32,6>)
    n171 = Multiply(x="Sin wave freq._y (Hz)", y=fxp<+/-,10,3> 2.0) -> (x*y=w430:fxp<+/-,41,9>)
    n172 = local read "Sin magnitude_y"() -> (w420:fxp<+/-,21,6>)
    n173 = local read "Sin magnitude_y"() -> (w413:fxp<+/-,21,6>)
    n174 = local read "Sin omega_y"() -> (w416:fxp<+/-,34,9>)
    n175 = Multiply(x=w430, y=w429) -> (x*y=w428:fxp<+/-,41,19>)
    n176 = Square(x=w416) -> (x^2=w415:fxp<+,34,18>)
    n177 = xnode "High Throughput Sine & Cosine"("x (pi)"=w428) -> ("sin(x)"=w410:fxp<+/-,16,2>, "cos(x)"=w418:fxp<+/-,16,2>)
    n178 = Multiply(x=w423, y=w422) -> (x*y=w421:fxp<+/-,34,9>)
    "Sin omega_y" <- w421
    n179 = Negate(x=w415) -> (-x=w414:fxp<+/-,35,19>)
    n180 = Multiply(x=w421, y=w420) -> (x*y=w419:fxp<+/-,33,15>)
    n181 = Multiply(x=w414, y=w413) -> (x*y=w412:fxp<+/-,34,20>)
    n182 = Multiply(x=w418, y=w419) -> (x*y=→"Dyr_sin_d":fxp<+/-,33,15>)
    n183 = Multiply(x="Sin magnitude_y", y=w410) -> (x*y=w426:fxp<+/-,37,8>)
    n184 = Multiply(x=w410, y=w412) -> (x*y=→"Dyr_sin_dd":fxp<+/-,35,20>)
    n185 = Add(x=w426, y="Sin offset_y") -> (x+y=→"Dyr_sin":fxp<+/-,37,8>)
    n186 = local read "Sin wave freq._p (Hz)"() -> (w387:fxp<+/-,32,6>)
    n187 = local read "Time now(s)"() -> (w405:fxp<+,52,14>)
    n188 = local read "Sin magnitude_p"() -> (w388:fxp<+/-,21,6>)
    n189 = local read "Sin magnitude_p"() -> (w390:fxp<+/-,21,6>)
    n190 = local read "Sin omega_p"() -> (w389:fxp<+/-,34,9>)
    n191 = Multiply(x="Sin wave freq._p (Hz)", y=fxp<+/-,10,3> 2.0) -> (x*y=w409:fxp<+/-,42,9>)
    n192 = Multiply(x=w409, y=w405) -> (x*y=w406:fxp<+/-,41,19>)
    n193 = Square(x=w389) -> (x^2=w401:fxp<+,34,18>)
    n194 = xnode "High Throughput Sine & Cosine"("x (pi)"=w406) -> ("sin(x)"=w392:fxp<+/-,16,2>, "cos(x)"=w397:fxp<+/-,16,2>)
    n195 = Multiply(x=w391, y=w387) -> (x*y=w404:fxp<+/-,34,9>)
    "Sin omega_p" <- w404
    n196 = Negate(x=w401) -> (-x=w400:fxp<+/-,35,19>)
    n197 = Multiply(x=w404, y=w388) -> (x*y=w403:fxp<+/-,33,15>)
    n198 = Multiply(x=w400, y=w390) -> (x*y=w399:fxp<+/-,35,19>)
    n199 = Multiply(x=w397, y=w403) -> (x*y=→"Dpr_sin_d":fxp<+/-,33,15>)
    n200 = Multiply(x=w392, y=w399) -> (x*y=→"Dpr_sin_dd":fxp<+/-,35,20>)
    n201 = Multiply(x="Sin magnitude_p", y=w392) -> (x*y=w395:fxp<+/-,37,8>)
    n202 = Add(x=w395, y="Sin offset_p") -> (x+y=→"Dpr_sin":fxp<+/-,37,8>)
  }
  n203 = while "Time reset" {
    shift-right: [w502] -> _
    shift-left: _ -> [w503]
    shift-right: [w497] -> _
    shift-left: _ -> [w498]
    stop <- FALSE stop-if-true
    n204 = local read "Stop motor_y"() -> (w504:bool)
    n205 = call "Tick Count3"() -> ("Tick Count(uSec)"=w502:u32)
    n206 = Subtract(x=w502, y=w503) -> (x-y=w501:u32)
    n207 = Add(x=w498, y=w501) -> (x+y=w500:u32)
    n208 = Select(t=u32 0, s=w504, f=w500) -> (s? t:f=w497:u32)
    n209 = To Fixed-Point(number=w497) -> (fixed-point=w496:fxp<+,32,32>)  [unwired: 1 in]
    n210 = Multiply(x=fxp<+,20,-18> 1.0000003385357559e-06, y=w496) -> (x*y=→"Time now(s)":fxp<+,52,14>)
  }
  n211 = while "Ini" {
    stop <- FALSE stop-if-true
    n212 = case shown="True" "Ini coe." {
      frame False {
      }
      frame True {
        w523 = i16 0 items=["Step", "Sine"] ("Command_p")
        w524 = i16 2 items=["Raw", "Avg.", "Avg. w. filter"] ("Strain selection_p")
        w525 = i16 0 items=["Step", "Sine"] ("Command_y")
        w526 = i16 2 items=["Raw", "Avg.", "Avg. w. filter"] ("Strain selection_y")
        w528 = fxp<+/-,25,-10> 5.851034075021744e-07  # S/F coeff_p
        w527 = fxp<+/-,25,-10> 1.0477961041033268e-06  # S/F coeff_y
        w534 = i16 0 items=["Backward", "Forward"] ("Drive mode")
        n213 = local write "Sin wave freq._y (Hz)"(fxp<+/-,32,6> 1.0 ("Sin wave freq. (Hz)")) -> ()
        n214 = local write "Sin magnitude_y"(fxp<+/-,22,7> 5.0 ("Sin magnitude")) -> ()
        n215 = local write "fy_tolorance"(fxp<+,22,6> 5.0 ("f_tolorance")) -> ()
        n216 = local write "Sin offset_y"(fxp<+/-,38,9> 0.0 ("Sin offset")) -> ()
        n217 = local write "Dyr_step"(fxp<+/-,22,7> 0.0 ("Dr")) -> ()
        n218 = local write "Kp_y"(fxp<+/-,36,9> 30.0 ("Kp")) -> ()
        n219 = local write "Kd_y"(fxp<+/-,36,9> 0.0 ("Kd")) -> ()
        n220 = local write "Kv_y"(fxp<+/-,22,8> 0.0 ("Kv")) -> ()
        n221 = local write "Bv_y"(fxp<+/-,22,8> 0.0 ("Bv")) -> ()
        n222 = local write "Ki_y"(fxp<+/-,36,9> 0.0 ("Ki")) -> ()
        n223 = local write "S/F coeff_p"(w528) -> ()
        n224 = local write "S/F coeff_y"(w527) -> ()
        n225 = local write "dFy_add"(FALSE ("dF_add")) -> ()
        n226 = local write "dFp_add"(FALSE ("dFp_add")) -> ()
        n227 = local write "Sin wave freq._p (Hz)"(fxp<+/-,32,6> 1.0 ("Sin wave freq._p (Hz)")) -> ()
        n228 = local write "Sin magnitude_p"(fxp<+/-,21,6> 5.0 ("Sin magnitude_p")) -> ()
        n229 = local write "fp_tolorance"(fxp<+,22,6> 5.0 ("fp_tolorance")) -> ()
        n230 = local write "Sin offset_p"(fxp<+/-,22,7> 0.0 ("Sin offset_p")) -> ()
        n231 = local write "Dpr_step"(fxp<+/-,22,7> 0.0 ("Dpr_step")) -> ()
        n232 = local write "Kp_p"(fxp<+/-,36,9> 30.0 ("Kp_p")) -> ()
        n233 = local write "Kd_p"(fxp<+/-,36,9> 0.0 ("Kd_p")) -> ()
        n234 = local write "Kv_p"(fxp<+/-,22,8> 0.0 ("Kv_p")) -> ()
        n235 = local write "Bv_p"(fxp<+/-,22,8> 0.0 ("Bv_p")) -> ()
        n236 = local write "Ki_p"(fxp<+/-,36,9> 0.0 ("Ki_p")) -> ()
        n237 = local write "Strain selection_p"(w524) -> ()
        n238 = local write "Strain selection_y"(w526) -> ()
        n239 = local write "Command_p"(w523) -> ()
        n240 = local write "Command_y"(w525) -> ()
        n241 = local write "Drive mode"(w534) -> ()
        n242 = local write "Dp_d_M_avg_Tc (uSec)"(u32 1000 ("D_d_M_avg_Tc (uSec)")) -> ()
        n243 = local write "Belt_mp"(fxp<+/-,6,6> 16.0 ("Belt_mp")) -> ()
        n244 = local write "Belt_my"(fxp<+/-,6,6> 16.0 ("Belt_my")) -> ()
        n245 = local write "Belt_op"(fxp<+/-,7,7> 22.0 ("Belt_op")) -> ()
        n246 = local write "Belt_oy"(fxp<+/-,7,7> 22.0 ("Belt_oy")) -> ()
      }
    }
  }
  n247 = while "FIFO" {
    stop <- FALSE stop-if-true
    n248 = flat-sequence {
      frame #0 {
        n249 = call "Loop Timer"("Count(uSec)"=u32 1000) -> ()  [unwired: 1 out]
      }
      frame #1 {
        n250 = local read "D_y(mm)"() -> (w560:fxp<+/-,32,7>)
        n251 = local read "Raw Strain_y"() -> (w559:fxp<+/-,36,4>)
        n252 = local read "Strain_y (Avg8)"() -> (w558:fxp<+/-,36,4>)
        n253 = local read "Strain_y (Avg8 w. f)"() -> (w557:fxp<+/-,36,8>)
        n254 = local read "Force_y"() -> (w553:fxp<+/-,32,10>)
        n255 = local read "Fy_dc"() -> (w555:fxp<+/-,32,10>)
        n256 = local read "D_p(mm)"() -> (w552:fxp<+/-,32,7>)
        n257 = local read "Raw Strain_p"() -> (w551:fxp<+/-,36,4>)
        n258 = local read "Strain_p (Avg8)"() -> (w550:fxp<+/-,36,4>)
        n259 = local read "Strain_p (Avg8 w. f)"() -> (w549:fxp<+/-,36,8>)
        n260 = local read "Force_p"() -> (w548:fxp<+/-,32,10>)
        n261 = local read "Dp_d (mm/s)"() -> (w547:fxp<+/-,36,13>)
        n262 = local read "Fp_dc"() -> (w546:fxp<+/-,32,10>)
        n263 = local read "Dy_d (T)"() -> (w554:fxp<+/-,36,13>)
        n264 = Build Array(w560, w559, w558, w557, w553, w554, w555, i16 0, w552, w551, w550, w549, w548, w547, w546, 0 ("element")) -> (w544:fxp<+/-,64,32>[])
        n265 = xnode ("FIFO Write")("Element"=w544, "Timeout"=0) -> ()  [unwired: 1 in, 2 out]
      }
    }
  }
  n266 = while "PID force controller_y" {
    stop <- FALSE stop-if-true
    n267 = local read "Force_y"() -> (w578:fxp<+/-,32,10>)
    n268 = local read "fyt_d"() -> (w562:fxp<+/-,36,18>)
    n269 = local read "Fr_y"() -> (w564:fxp<+/-,32,10>)
    n270 = xnode "High Throughput Subtract"("x"=w564, "y"=w578) -> ("x-y"=w577:fxp<+/-,33,11>)
    "fy_tilde" <- w577
    n271 = Absolute Value(x=w577) -> (abs(x)=w568:fxp<+,33,11>)
    n272 = local read "fyt_i"() -> (w563:fxp<+/-,36,16>)
    n273 = xnode ("High Throughput Multiply")("x"="Kp_y", "y"=w577) -> ("x*y"=w575:fxp<+/-,64,20>)
    n274 = xnode ("High Throughput Multiply")("x"="Kd_y", "y"=w562) -> ("x*y"=w574:fxp<+/-,64,27>)
    n275 = xnode ("High Throughput Add")("x"=w575, "y"=w574) -> ("x+y"=w571:fxp<+/-,64,28>)
    n276 = xnode ("High Throughput Multiply")("x"="Ki_y", "y"=w563) -> ("x*y"=w572:fxp<+/-,64,25>)
    n277 = Greater?(x=w568, y="fy_tolorance") -> (0:w566:bool)
    n278 = xnode ("High Throughput Add")("x"=w571, "y"=w572) -> ("x+y"=w570:fxp<+/-,64,29>)
    n279 = Select(t=w570, s=w566, f=fxp<+/-,51,14> 0.0) -> (s? t:f=→"Fy_PID":fxp<+/-,64,29>)
  }
  n280 = while "Encoder_y" {
    shift-right: [w595] -> _
    shift-left: _ -> [w596]
    shift-right: [w597] -> _
    shift-left: _ -> [w598]
    shift-right: [w590] -> _
    shift-left: _ -> [w594]
    stop <- FALSE stop-if-true
    w586 = fxp<+/-,20,-5> 0.002499997615814209  # L/800
    n281 = xnode "FPGA I/O Node"() -> ("Mod4/DI3"=w593:bool, "Mod4/DI4"=w592:bool)  [unwired: 2 in, 2 out]
    n282 = local read "Belt_my"() -> (w585:fxp<+/-,6,6>)
    n283 = local read "Belt_oy"() -> (w583:fxp<+/-,7,7>)
    n284 = call "encoder_sub.vi"("A_pre"=w596, "B_pre"=w598, "Encoder Position_pre"=w594, "A input"=w593, "Encoder Position Reset"="Encoder reset_y", "B input"=w592) -> ("A"=w595:bool, "B"=w597:bool, "Encoder Position (Counts)"=w590:i32)  [unwired: 19 in]
    "Encoder Position_y" <- w590
    n285 = Multiply(x=w586, y=w585) -> (x*y=w584:fxp<+/-,26,1>)
    n286 = To Fixed-Point(number=w590) -> (fixed-point=w589:fxp<+/-,32,32>)  [unwired: 1 in]
    n287 = Divide(x=w584, y=w583) -> (x/y=w582:fxp<+/-,33,1>)
    n288 = xnode ("High Throughput Multiply")("x"=w589, "y"=w582) -> ("x*y"=→"D_y(mm)":fxp<+/-,64,33>)
    n289 = xnode ("High Throughput Multiply")("x"=w589, "y"=fxp<+/-,16,1> 0.125) -> ("x*y"=→"rad_y(NrTheta)":fxp<+/-,48,33>)
  }
  n290 = for {
    N: w5 -> [_]
    tunnel: [w601] -> w4 mode=indexing
    tunnel: [w600] -> w3 mode=indexing
    tunnel: ["Dy_d_M_avg_Tc (uSec)"] -> w2
    n291 = local read "Encoder Position_y"() -> (w600:i32)
    n292 = call "Wait3"("Count(uSec)"="Dy_d_M_avg_Tc (uSec)") -> ("Tick Count(uSec)"=w601:u32)
  }
  n293 = for {
    N: w8 -> [_]
    tunnel: ["Dp_d_M_avg_Tc (uSec)"] -> w1
    tunnel: [w603] -> w7 mode=indexing
    tunnel: [w602] -> w6 mode=indexing
    n294 = local read "Encoder Position_p"() -> (w602:i32)
    n295 = call "Wait2"("Count(uSec)"="Dp_d_M_avg_Tc (uSec)") -> ("Tick Count(uSec)"=w603:u32)
  }
  n296 = local read "Dy_d_M_avg_Tc (uSec)"() -> ()  [unwired: 1 out]
  n297 = while "Omega_y (Mavg)" {
    tunnel: w5 -> [w621]
    shift-right: [w619] -> _
    shift-left: w4 -> [w624]
    shift-right: [w618] -> _
    shift-left: w3 -> [w620]
    shift-right: [w606] -> _
    shift-left: _ -> [w617]
    tunnel: w2 -> [w605]
    stop <- FALSE stop-if-true
    w610 = fxp<+/-,32,0> 0.3183098859153688  # L/2/pi
    n298 = call "Tick Count6"() -> ("Tick Count(uSec)"=w625:u32)
    n299 = Index Array(array=w624, index=0) -> (element=w623:u32)
    n300 = Index Array(array=w620, index=0) -> (element=w622:i32)
    n301 = Multiply(x=w621, y=w605) -> (x*y=w627:i32)
    n302 = Add(x=w627, y=w623) -> (x+y=w626:u32)
    n303 = Greater Or Equal?(x=w625, y=w626) -> (x >= y?=w616:bool)
    n304 = case shown="True" w616 {
      tunnel: w625 -> [_ w648]
      tunnel: w621 -> [_ w645]
      tunnel: w624 -> [w632 w647]
      tunnel: w623 -> [_ w646]
      tunnel: w622 -> [_ w639]
      tunnel: w620 -> [w631 w644]
      tunnel: [w630 w636] -> w606
      tunnel: [w632 w635] -> w619
      tunnel: [w631 w634] -> w618
      tunnel: w617 -> [w630 _]
      frame False {
      }
      frame True {
        n305 = local read "Encoder Position_y"() -> (w638:i32)
        n306 = Subtract(x=w648, y=w646) -> (x-y=w649:u32)
        n307 = Subtract(x=w638, y=w639) -> (x-y=w643:i32)
        n308 = Insert Into Array(array=w647, new element=w648) -> (w651:u32[])  [unwired: 1 in]
        n309 = Insert Into Array(array=w644, index=w645, new element=w638) -> (w652:i32[])
        n310 = Multiply(x=w643, y=2500) -> (x*y=w641:i32)
        n311 = To Fixed-Point(number=w649) -> (fixed-point=w637:fxp<+,32,32>)  [unwired: 1 in]
        n312 = To Fixed-Point(number=w641) -> (fixed-point=w640:fxp<+/-,32,32>)  [unwired: 1 in]
        n313 = Delete From Array(array=w651, length=1, index=0) -> (array with subset deleted=w635:u32[])  [unwired: 1 out]
        n314 = Delete From Array(array=w652, length=1, index=0) -> (array with subset deleted=w634:i32[])  [unwired: 1 out]
        n315 = Divide(x=w640, y=w637) -> (x/y=w636:fxp<+/-,64,32>)
      }
    }
    n316 = local read "Belt_my"() -> (w614:fxp<+/-,6,6>)
    n317 = Multiply(x=fxp<+/-,27,3> 3.1415926218032837, y=w606) -> (x*y=w609:fxp<+/-,64,35>)
    "omega_y (Mavg)" <- w609
    n318 = local read "Belt_oy"() -> (w613:fxp<+/-,7,7>)
    n319 = Multiply(x=w609, y=w610) -> (x*y=w611:fxp<+/-,64,35>)
    n320 = Multiply(x=w611, y=w614) -> (x*y=w612:fxp<+/-,64,41>)
    n321 = Divide(x=w612, y=w613) -> (x/y=→"Dy_d (Mavg)":fxp<+/-,64,42>)
  }
  n322 = while "Omega_p (Mavg)" {
    tunnel: w8 -> [w678]
    shift-right: [w676] -> _
    shift-left: w7 -> [w681]
    shift-right: [w675] -> _
    shift-left: w6 -> [w677]
    shift-right: [w674] -> _
    shift-left: _ -> [w673]
    tunnel: w1 -> [w671]
    stop <- FALSE stop-if-true
    w658 = fxp<+/-,32,0> 0.3183098859153688  # L/2/pi
    w668 = fxp<+,32,0> 0.1953125  # 800/4096
    n323 = call "Tick Count5"() -> ("Tick Count(uSec)"=w682:u32)
    n324 = Index Array(array=w681, index=0) -> (element=w680:u32)
    n325 = Index Array(array=w677, index=0) -> (element=w679:i32)
    n326 = Multiply(x=w678, y=w671) -> (x*y=w684:i32)
    n327 = Add(x=w684, y=w680) -> (x+y=w683:u32)
    n328 = Greater Or Equal?(x=w682, y=w683) -> (x >= y?=w672:bool)
    n329 = case shown="True" w672 {
      tunnel: w682 -> [_ w705]
      tunnel: w678 -> [_ w702]
      tunnel: w681 -> [w689 w704]
      tunnel: w680 -> [_ w703]
      tunnel: w679 -> [_ w696]
      tunnel: w677 -> [w688 w701]
      tunnel: [w687 w693] -> w674
      tunnel: [w689 w692] -> w676
      tunnel: [w688 w691] -> w675
      tunnel: w673 -> [w687 _]
      frame False {
      }
      frame True {
        n330 = local read "Encoder Position_p"() -> (w695:i32)
        n331 = Subtract(x=w705, y=w703) -> (x-y=w706:u32)
        n332 = Subtract(x=w695, y=w696) -> (x-y=w700:i32)
        n333 = Insert Into Array(array=w704, new element=w705) -> (w708:u32[])  [unwired: 1 in]
        n334 = Insert Into Array(array=w701, index=w702, new element=w695) -> (w709:i32[])
        n335 = Multiply(x=w700, y=2500) -> (x*y=w698:i32)
        n336 = To Fixed-Point(number=w706) -> (fixed-point=w694:fxp<+,32,32>)  [unwired: 1 in]
        n337 = To Fixed-Point(number=w698) -> (fixed-point=w697:fxp<+/-,32,32>)  [unwired: 1 in]
        n338 = Delete From Array(array=w708, length=1, index=0) -> (array with subset deleted=w692:u32[])  [unwired: 1 out]
        n339 = Delete From Array(array=w709, length=1, index=0) -> (array with subset deleted=w691:i32[])  [unwired: 1 out]
        n340 = Divide(x=w697, y=w694) -> (x/y=w693:fxp<+/-,64,32>)
      }
    }
    n341 = local read "Mag. factor"() -> (w664:fxp<+/-,20,3>)
    n342 = local read "Mag. encoder_p"() -> (w669:bool)
    n343 = Multiply(x=w664, y=w668) -> (x*y=w670:fxp<+/-,52,3>)
    n344 = Select(t=w670, s=w669, f=fxp<+/-,52,3> 1.0) -> (s? t:f=w665:fxp<+/-,52,3>)
    n345 = Multiply(x=w665, y=w674) -> (x*y=w666:fxp<+/-,64,34>)
    n346 = local read "Belt_mp"() -> (w662:fxp<+/-,6,6>)
    n347 = Multiply(x=fxp<+/-,27,3> 3.1415926218032837, y=w666) -> (x*y=w657:fxp<+/-,64,37>)
    "omega_p (Mavg)" <- w657
    n348 = local read "Belt_op"() -> (w661:fxp<+/-,7,7>)
    n349 = Multiply(x=w657, y=w658) -> (x*y=w659:fxp<+/-,64,37>)
    n350 = Multiply(x=w659, y=w662) -> (x*y=w660:fxp<+/-,64,43>)
    n351 = Divide(x=w660, y=w661) -> (x/y=→"Dp_d (Mavg)":fxp<+/-,64,44>)
  }
  n352 = while "Quadrature drive_p" {
    stop <- FALSE stop-if-true
    n353 = local read "dFp_PID"() -> (w713:fxp<+/-,36,18>)
    n354 = local read "omega_p (rad/s)"() -> (w719:fxp<+/-,36,13>)
    n355 = local read "Fp_PID"() -> (w714:fxp<+/-,36,16>)
    n356 = Select(t=w713, s="dFp_add", f=fxp<+,1,1> 0.0) -> (s? t:f=w717:fxp<+/-,36,18>)
    n357 = call "Oriental_step_motor_PKP225.vi"("F_Threshold"=fxp<+,12,12> 10.0, "dFmr"=w717, "omega"=w719, "Fmr"=w714) -> ("vq_F"=→"vq_p_F":fxp<+/-,20,5>, "vd_F"=→"vd_p_F":fxp<+/-,20,5>)  [unwired: 6 in]
  }
  n358 = while "PID force controller_p" {
    stop <- FALSE stop-if-true
    n359 = local read "Force_p"() -> (w734:fxp<+/-,32,10>)
    n360 = local read "fpt_d"() -> (w725:fxp<+/-,36,18>)
    n361 = local read "Fr_p"() -> (w735:fxp<+/-,32,10>)
    n362 = xnode "High Throughput Subtract"("x"=w735, "y"=w734) -> ("x-y"=w726:fxp<+/-,33,11>)
    "fp_tilde" <- w726
    n363 = local read "fpt_i"() -> (w723:fxp<+/-,34,18>)
    n364 = xnode ("High Throughput Multiply")("x"="Kp_p", "y"=w726) -> ("x*y"=w724:fxp<+/-,64,20>)
    n365 = xnode ("High Throughput Multiply")("x"="Kd_p", "y"=w725) -> ("x*y"=w740:fxp<+/-,64,27>)
    n366 = Absolute Value(x=w726) -> (abs(x)=w733:fxp<+,33,11>)
    n367 = xnode ("High Throughput Add")("x"=w724, "y"=w740) -> ("x+y"=w738:fxp<+/-,64,28>)
    n368 = xnode ("High Throughput Multiply")("x"="Ki_p", "y"=w723) -> ("x*y"=w739:fxp<+/-,64,27>)
    n369 = xnode ("High Throughput Add")("x"=w738, "y"=w739) -> ("x+y"=w729:fxp<+/-,64,29>)
    n370 = Greater?(x=w733, y="fp_tolorance") -> (0:w730:bool)
    n371 = Select(t=w729, s=w730, f=fxp<+,1,1> 0.0) -> (s? t:f=→"Fp_PID":fxp<+/-,64,29>)
  }
  n372 = while "PD position controller_p" {
    stop <- FALSE stop-if-true
    n373 = local read "Drive mode"() -> (w743:i16)
    n374 = case shown="1" w743 {
      tunnel: [fxp<+/-,62,19> 0.0 w746] -> w742
      frame 0, Default {
        # "Backward"
      }
      frame 1 {
        # "Forward"
        n375 = local read "D_p(mm)"() -> (w753:fxp<+/-,32,7>)
        n376 = local read "Dp_error_d"() -> (w745:fxp<+/-,33,8>)
        n377 = local read "Dpr_for"() -> (w752:fxp<+/-,22,7>)
        n378 = Subtract(x=w752, y=w753) -> (x-y=w751:fxp<+/-,24,8>)
        "Dp_error" <- w751
        n379 = Multiply(x=w751, y="Kv_p") -> (x*y=w748:fxp<+/-,34,16>)
        n380 = Multiply(x=w745, y="Bv_p") -> (x*y=w747:fxp<+/-,55,16>)
        n381 = Add(x=w748, y=w747) -> (x+y=w746:fxp<+/-,56,17>)
      }
    }
    "Fr_p" <- w742
  }
  n382 = while "All switch" {
    stop <- FALSE stop-if-true
    n383 = case shown="True" "Encoder reset" {
      frame False {
        n384 = local write "Encoder reset_p"(FALSE ("Encoder reset_p")) -> ()
        n385 = local write "Encoder reset_y"(FALSE ("Encoder reset_y")) -> ()
      }
      frame True {
        n386 = flat-sequence {
          frame #0 {
            n387 = local write "Encoder reset_p"(TRUE ("Encoder reset_p")) -> ()
          }
          frame #1 {
            n388 = local write "Encoder reset_y"(TRUE ("Encoder reset_y")) -> ()
            n389 = local write "Encoder reset_p"(FALSE ("Encoder reset_p")) -> ()
          }
          frame #2 {
            n390 = local write "Encoder reset_y"(FALSE ("Encoder reset_y")) -> ()
          }
        }
      }
    }
  }
  n391 = while "Derivative" {
    stop <- FALSE stop-if-true
    n392 = local read "Dpr_sin_dd"() -> (w770:fxp<+/-,35,20>)
    n393 = local read "Stop motor_y"() -> (w776:bool)
    n394 = local read "Dyr_sin_dd"() -> (w778:fxp<+/-,35,20>)
    n395 = local read "Dpr_sin_d"() -> (w772:fxp<+/-,33,15>)
    n396 = local read "Stop motor_p"() -> (w768:bool)
    n397 = local read "Dyr_sin_d"() -> (w781:fxp<+/-,33,15>)
    n398 = local read "Dp_error"() -> (w773:fxp<+/-,22,7>)
    n399 = local read "Dy_error"() -> (w782:fxp<+/-,22,7>)
    n400 = local read "Dp_dd"() -> (w771:fxp<+/-,36,25>)
    n401 = local read "Dy_dd"() -> (w779:fxp<+/-,36,25>)
    n402 = Subtract(x=w781, y=w782) -> (x-y=w780:fxp<+/-,34,16>)
    n403 = Subtract(x=w778, y=w779) -> (x-y=w777:fxp<+/-,41,26>)
    n404 = Subtract(x=w772, y=w773) -> (x-y=w765:fxp<+/-,34,16>)
    n405 = Subtract(x=w770, y=w771) -> (x-y=w769:fxp<+/-,41,26>)
    n406 = Select(t=fxp<+,1,1> 0.0, s=w776, f=w780) -> (s? t:f=→"Dy_error_d":fxp<+/-,34,16>)
    n407 = Select(t=fxp<+/-,64,49> 0.0, s=w776, f=w777) -> (s? t:f=→"Dy_error_dd":fxp<+/-,64,49>)
    n408 = Select(t=fxp<+,1,1> 0.0, s=w768, f=w765) -> (s? t:f=→"Dp_error_d":fxp<+/-,34,16>)
    n409 = Select(t=fxp<+/-,41,26> 0.0, s=w768, f=w769) -> (s? t:f=→"Dp_error_dd":fxp<+/-,41,26>)
  }
  n410 = while "ft_d" {
    stop <- FALSE stop-if-true
    n411 = local read "Dy_error_dd"() -> (w800:fxp<+/-,36,16>)
    n412 = local read "Dp_error_dd"() -> (w791:fxp<+/-,36,16>)
    n413 = local read "Dy_error_d"() -> (w802:fxp<+/-,33,8>)
    n414 = local read "Dp_error_d"() -> (w793:fxp<+/-,33,8>)
    n415 = local read "Kv_p"() -> (w794:fxp<+/-,22,8>)
    n416 = local read "Bv_p"() -> (w792:fxp<+/-,22,8>)
    n417 = local read "Kv_y"() -> (w803:fxp<+/-,22,8>)
    n418 = local read "Bv_y"() -> (w801:fxp<+/-,22,8>)
    n419 = local read "Force_y"() -> (w796:fxp<+/-,32,10>)
    n420 = Multiply(x=w802, y=w803) -> (x*y=w798:fxp<+/-,55,16>)
    n421 = Multiply(x=w800, y=w801) -> (x*y=w799:fxp<+/-,58,24>)
    n422 = Multiply(x=w793, y=w794) -> (x*y=w789:fxp<+/-,55,16>)
    n423 = Multiply(x=w791, y=w792) -> (x*y=w790:fxp<+/-,58,24>)
    n424 = local read "Force_p"() -> (w787:fxp<+/-,32,10>)
    n425 = Add(x=w798, y=w799) -> (x+y=w797:fxp<+/-,63,24>)
    n426 = Add(x=w789, y=w790) -> (x+y=w788:fxp<+/-,63,24>)
    n427 = Subtract(x=w797, y=w796) -> (x-y=→"fyt_d":fxp<+/-,63,24>)
    n428 = Subtract(x=w788, y=w787) -> (x-y=→"fpt_d":fxp<+/-,63,24>)
  }
  n429 = while "Encoder_p" {
    shift-right: [w825] -> _
    shift-left: _ -> [w826]
    shift-right: [w827] -> _
    shift-left: _ -> [w828]
    shift-right: [w821] -> _
    shift-left: _ -> [w829]
    stop <- FALSE stop-if-true
    w806 = fxp<+,32,0> 0.1953125  # 800/4096
    w816 = fxp<+/-,20,-5> 0.002499997615814209  # L/800
    w820 = fxp<+/-,16,1> 0.125  # 2pi*50/800
    n430 = xnode "FPGA I/O Node"() -> ("Mod4/DI0"=w823:bool, "Mod4/DI1"=w824:bool)  [unwired: 2 in, 2 out]
    n431 = local read "Belt_mp"() -> (w815:fxp<+/-,6,6>)
    n432 = local read "Belt_op"() -> (w813:fxp<+/-,7,7>)
    n433 = call "encoder_sub.vi"("A_pre"=w826, "B_pre"=w828, "Encoder Position_pre"=w829, "A input"=w823, "Encoder Position Reset"="Encoder reset_p", "B input"=w824) -> ("A"=w825:bool, "B"=w827:bool, "Encoder Position (Counts)"=w821:i32)  [unwired: 19 in]
    "Encoder Position_p" <- w821
    n434 = Multiply(x=w806, y="Mag. factor") -> (x*y=w812:fxp<+/-,52,3>)
    n435 = To Fixed-Point(number=w821) -> (fixed-point=w808:fxp<+/-,32,32>)  [unwired: 1 in]
    n436 = Multiply(x=w816, y=w815) -> (x*y=w814:fxp<+/-,26,1>)
    n437 = Select(t=w812, s="Mag. encoder_p", f=fxp<+/-,20,3> 1.0) -> (s? t:f=w807:fxp<+/-,52,3>)
    n438 = Divide(x=w814, y=w813) -> (x/y=w804:fxp<+/-,33,1>)
    n439 = Multiply(x=w807, y=w808) -> (x*y=w805:fxp<+/-,64,35>)
    n440 = xnode ("High Throughput Multiply")("x"=w805, "y"=w820) -> ("x*y"=→"rad_p(NrTheta)":fxp<+/-,64,36>)
    n441 = xnode ("High Throughput Multiply")("x"=w804, "y"=w805) -> ("x*y"=→"D_p(mm)":fxp<+/-,64,36>)
  }
  n442 = while "Omega_p(T method)" {
    shift-right: [w852] -> _
    shift-left: _ -> [w850]
    shift-right: [w832] -> _
    shift-left: _ -> [w851]
    shift-right: [w847] -> _
    shift-left: _ -> [w849]
    stop <- FALSE stop-if-true
    w833 = fxp<+,32,0> 0.1953125  # 800/4096
    w843 = fxp<+/-,32,0> 0.3183098859153688  # L/2/pi
    n443 = call "Tick Count4"() -> ("Tick Count(Ticks)"=w848:u32)
    n444 = local read "Encoder Position_p"() -> (w852:i32)
    n445 = local read "Mag. factor"() -> (w834:fxp<+/-,20,3>)
    n446 = local read "Mag. encoder_p"() -> (w835:bool)
    n447 = call "omega_sub_Encoder_800ppr.vi"("mt0"="mt0_omega_p", "omega_pre"=w851, "ticks_m_pre"=w849, "ticks"=w848, "count_pre"=w850, "count"=w852) -> ("ticks_m"=w847:u32, "mt"=→"mt_omega_p":u32, "omega"=w832:fxp<+/-,36,13>)  [unwired: 3 in]
    n448 = Multiply(x=w834, y=w833) -> (x*y=w836:fxp<+/-,52,3>)
    n449 = Multiply(x=w843, y="Belt_mp") -> (x*y=w841:fxp<+/-,38,6>)
    n450 = Select(t=w836, s=w835, f=fxp<+,2,1> 1.0) -> (s? t:f=w838:fxp<+/-,52,3>)
    n451 = Divide(x=w841, y="Belt_op") -> (x/y=w839:fxp<+/-,20,1>)
    n452 = Multiply(x=w832, y=w838) -> (x*y=w831:fxp<+/-,64,15>)
    "omega_p (T)" <- w831
    n453 = xnode ("High Throughput Multiply")("x"=w839, "y"=w831) -> ("x*y"=→"Dp_d (T)":fxp<+/-,64,16>)
  }
  n454 = xnode "FPGA I/O Node"("error in"=w9, "Mod6/Stop"=TRUE) -> ()  [unwired: 1 in, 2 out]
